vi "Write Timestamp NVM.vi"(0 "Session Handle in":T1, 5 "Serial Number":string, 11 "error in (no error)":errorcluster) -> (4 "Session Handle out":T1, 15 "error out":errorcluster)   [LabVIEW 2015, in "Gas.lvclass"]
uses:
  Gas.lvclass
  Typedefs/Session Handle.ctl
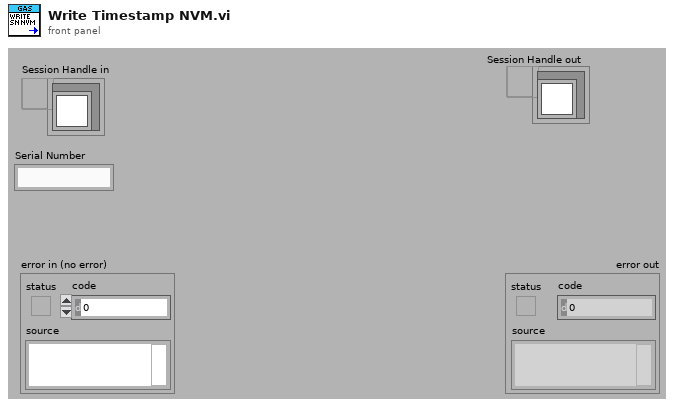
[diagram p1: front panel]
types:
  T1 = typedef "Gas.lvclass/Session Handle.ctl" = refnum<data-value>
  T2 = typedef "XNET Frame CAN.ctl" = cluster{"timestamp":timestamp, "payload":u8[], "identifier":u32, "type":T3, "extended?":bool, "echo?":bool}
  T3 = typedef "XNET Frame Type CAN.ctl" = u8
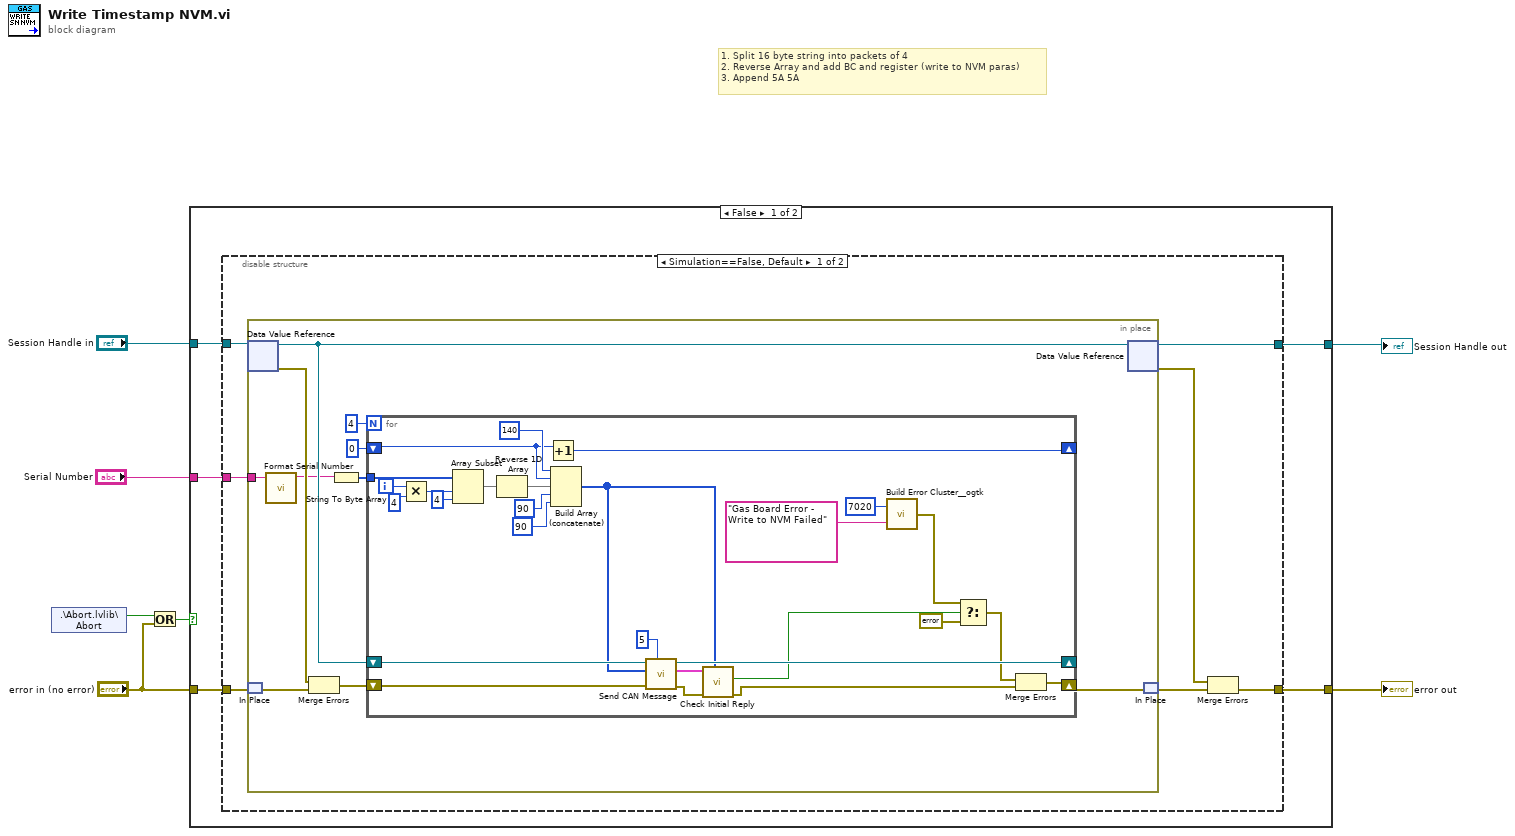
[diagram p0: block diagram]
diagram:
  # "1. Split 16 byte string into packets of 4\n2. Reverse Array and add BC and register (write to NVM paras)\n3. Append 5A 5A"
  n1 = shared-variable ".\\Abort.lvlib\\Abort"() -> (w4:bool)  [unwired: 1 in, 1 out]
  n2 = Or(x=w4, y="error in (no error)") -> (x .or. y?=w2:bool)
  n3 = case shown="False" w2 {
    tunnel: [w12 w60] -> w6
    tunnel: [w11 w59] -> w5
    tunnel: "Session Handle in" -> [w10 w60]
    tunnel: "error in (no error)" -> [w9 w59]
    tunnel: "Serial Number" -> [w8 _]
    frame False {
      n4 = disable-structure shown="Simulation==False, Default" {
        disable-tunnel: [w19 w58] -> w12
        disable-tunnel: [w16 w57] -> w11
        disable-tunnel: w10 -> [w15 w58]
        disable-tunnel: w9 -> [w14 w57]
        disable-tunnel: w8 -> [w13 _]
        frame condition #0 (active) {
          n5 = in-place {
            in-place-border: w13 -> [w21]
            n6 = in-place-dvr #1(w15) -> (w23:refnum<class "Gas.lvclass">, w29:errorcluster)
            n7 = in-place-match #2(w14) -> (w28:errorcluster)
            n8 = call "Format Serial Number.vi"("Serial Number"=w21) -> ("Serial Number Out"=w20:string)  [unwired: 10 in]
            n9 = Merge Errors(w29, w28) -> (w24:errorcluster)
            n10 = String To Byte Array(string=w20) -> (unsigned byte array=w27:u8[])
            n11 = for {
              N: 4 -> [_]
              tunnel: w27 -> [w56]
              shift-right: [w46] -> _
              shift-left: u8 0 -> [w45]
              shift-right: [w33] -> w22
              shift-left: w24 -> [w43]
              shift-right: [w41] -> _
              shift-left: w23 -> [w42]
              i -> [w55]
              n12 = Multiply(x=w55, y=4) -> (x*y=w53:i32)
              n13 = Array Subset(array=w56, index=w53, length=4) -> (w51:u8[])
              n14 = Reverse 1D Array(array=w51) -> (reversed array=w49:u8[])
              n15 = Increment(x=w45) -> (x+1=w46:u8)
              n16 = Build Array (concatenate)(u8 140, w45, w49, u8 90, u8 90) -> (w39:u8[])
              n17 = call "Send CAN Message.vi"("Number of Retries"=5, "error in (no error)"=w43, "payload"=w39, "Gas In"=w42) -> ("error out"=w31:errorcluster, "Reply"=w40:T2[], "Gas Out"=w41:refnum<class "Gas.lvclass">)  [unwired: 5 in]
              n18 = call "Check Initial Reply.vi"("Write Message"=w39, "error in (no error)"=w31, "Reply"=w40) -> ("error out"=w30:errorcluster, "Message Failed?"=w38:bool)  [unwired: 5 in, 2 out]
              n19 = call <userlib>:"Build Error Cluster__ogtk.vi"("String to Prepend to source (\"\")"="Gas Board Error - Write to NVM Failed" ("string"), "code"=7020) -> ("error out"=w35:errorcluster)
              n20 = Select(t=w35, s=w38, f=errorcluster {"status"=FALSE, "code"=0, "source"=""}) -> (s? t:f=w32:errorcluster)
              n21 = Merge Errors(w32, w30) -> (w33:errorcluster)
            }
            n22 = in-place-dvr #1(w23) -> (w19:T1, w17:errorcluster)
            n23 = in-place-match #2(w22) -> (w18:errorcluster)
          }
          n24 = Merge Errors(w17, w18) -> (w16:errorcluster)
        }
        frame condition #1 {
        }
      }
    }
    frame True {
    }
  }
  "Session Handle out" <- w6
  "error out" <- w5
